vi "CreateDirectory.vi"(9 "path":string, 10 "Ftp":refnum<k24>, 11 "error in":errorcluster) -> (3 "error out":errorcluster)   [LabVIEW 2024, in "UnderAutomation.Fanuc.lvlib"]
uses:
  UnderAutomation.Fanuc.lvlib
  C:/Users/fg/Documents/Fanuc.vi/LabVIEW_2024/UnderAutomation.Fanuc/lib/UnderAutomation.Fanuc.dll
  lib/UnderAutomation.Fanuc.dll
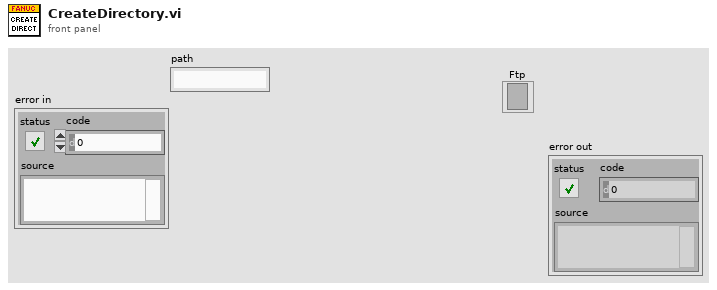
[diagram p1: front panel]
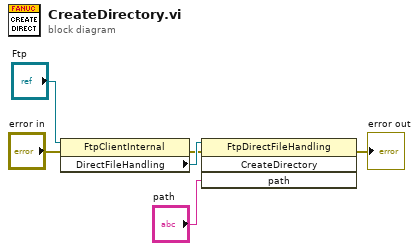
[diagram p0: block diagram]
diagram:
  n1 = property class="FtpClientInternal"(reference="Ftp", error in="error in") -> (error out=w1:errorcluster, "DirectFileHandling"=w4:refnum<k24>)  [unwired: 1 out]
  n2 = invoke class="FtpDirectFileHandling" method="CreateDirectory"(reference=w4, error in=w1, "path"="path") -> (error out=→"error out":errorcluster)  [unwired: 1 in, 3 out]
